vi "DC filter(移動平均濾波器 Sub VI).vi"(1 "當前迴圈計數(i)":i32, 2 "平均時間":dbl=2000.0, 3 "取樣頻率(Hz)":i32=2000, 4 "input signal":dbl) -> (0 "DC filter output":dbl)   [LabVIEW 2010]
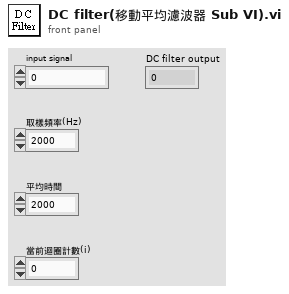
[diagram p1: front panel]
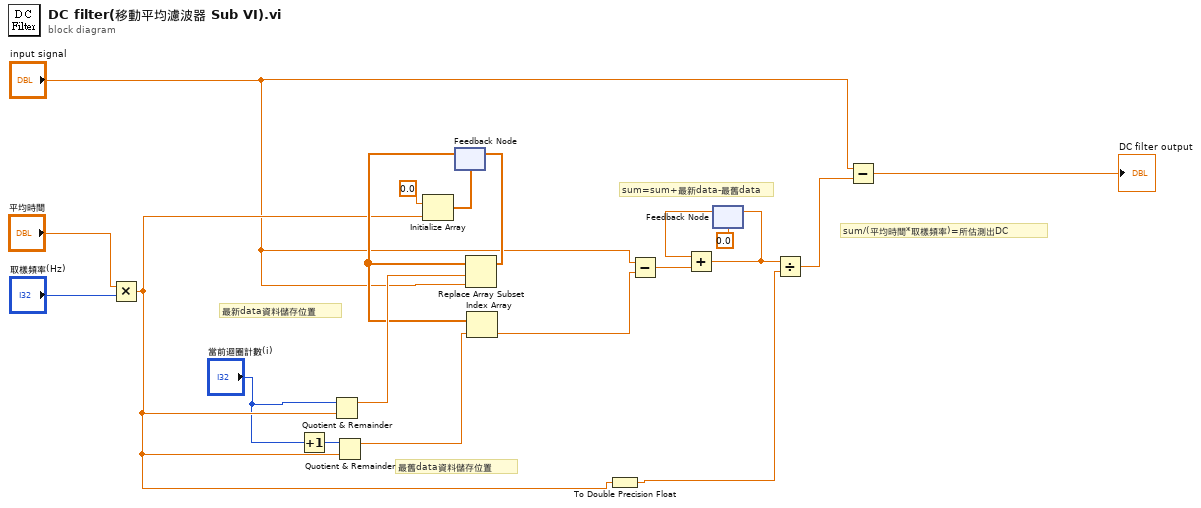
[diagram p0: block diagram]
diagram:
  # "sum/(平均時間*取樣頻率)=所估測出DC"
  # "sum=sum+最新data-最舊data"
  # "最新data資料儲存位置"
  # "最舊data資料儲存位置"
  n1 = Multiply(x="平均時間", y="取樣頻率(Hz)") -> (x*y=w5:dbl)
  n2 = Increment(x="當前迴圈計數(i)") -> (x+1=w19:i32)
  n3 = Quotient & Remainder(x="當前迴圈計數(i)", y=w5) -> (x-y*floor(x/y)=w18:dbl)  [unwired: 1 out]
  n4 = Quotient & Remainder(x=w19, y=w5) -> (x-y*floor(x/y)=w17:dbl)  [unwired: 1 out]
  n5 = Initialize Array(0.0 ("element"), w5) -> (w7:dbl[])
  n6 = feedback #1(w7) -> (w9:dbl[])
  n7 = Replace Array Subset(array=w9, new element="input signal", index=w18) -> (w10:dbl[])
  n8 = feedback-in #1(w10) -> ()
  n9 = Index Array(array=w9, index=w17) -> (element=w16:dbl)
  n10 = To Double Precision Float(number=w5) -> (double precision float=w11:dbl)
  n11 = Subtract(x="input signal", y=w16) -> (x-y=w15:dbl)
  n12 = feedback #2(0.0) -> (w14:dbl)
  n13 = Add(x=w14, y=w15) -> (x+y=w12:dbl)
  n14 = feedback-in #2(w12) -> ()
  n15 = Divide(x=w12, y=w11) -> (x/y=w3:dbl)
  n16 = Subtract(x="input signal", y=w3) -> (x-y=→"DC filter output":dbl)
